vi "Set Child.vi"(6 "Index in":i32, 8 "error in (no error)":errorcluster, 10 "Child":refnum<class "CConfig Object.lvclass">, 11 "Composite Object in":refnum<class "CConfig Object.lvclass">) -> (0 "error out":errorcluster, 3 "Composite Object out":refnum<class "CConfig Object.lvclass">)   [LabVIEW 2013, in "CConfig Object.lvclass"]
doc: "Copyright 2018, Carya Automatisering, Wiebe Walstra."
uses:
  CConfig Object.lvclass
  CConfig Object.lvclass/CConfig Object.ctl
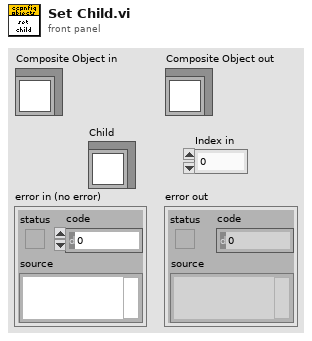
[diagram p1: front panel]
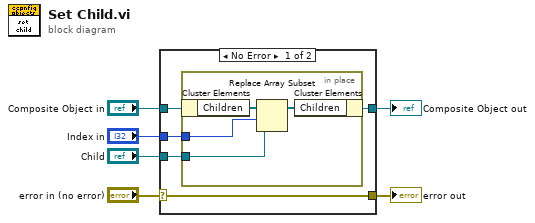
[diagram p0: block diagram]
diagram:
  n1 = case shown="No Error" "error in (no error)" {
    selector: "error in (no error)" -> [w11 w17]
    tunnel: [w11 w17] -> w5
    tunnel: [w9 w16] -> w1
    tunnel: "Composite Object in" -> [w10 w16]
    tunnel: "Index in" -> [w8 _]
    tunnel: "Child" -> [w7 _]
    frame No Error {
      n2 = in-place {
        in-place-border: w8 -> [w13]
        in-place-border: w7 -> [w12]
        n3 = in-place-cluster #1(w10) -> ("Children"=w15:refnum<class>[])
        n4 = Replace Array Subset(array=w15, new element=w12, index=w13) -> (w14:refnum<class>[])
        n5 = in-place-cluster #1("Children"=w14) -> (w9:refnum<class "CConfig Object.lvclass">)
      }
    }
    frame Error {
    }
  }
  "error out" <- w5
  "Composite Object out" <- w1
